vi "Exit Initialize (User).vi"(8 "error in":errorcluster, 11 "Node in":refnum<class "BLS Cycler Template.lvclass">) -> (0 "error out":errorcluster, 3 "Node out":refnum<class "BLS Cycler Template.lvclass">)   [LabVIEW 2023, in "BLS Cycler Template.lvlib" / "BLS Cycler Template.lvclass"]
uses:
  BLS Cycler Template.lvclass
  BLS Cycler Template.lvclass/BLS Cycler Template.ctl
  bls-capabilities/src/Capabilities/High Level Capabilities/Cycler/Cycler.lvclass
  <vilib>/ADAS Replay HIL/Template Node/Plugin/Template Node/Template Node.lvclass
  C:/Program Files/National Instruments/LabVIEW 2023/vi.lib/ADAS Replay HIL/Template Node/Plugin/Template Node/Template Node.lvclass
  C:/Program Files/National Instruments/ADAS Replay HIL/EVO SDK/Linux RT/evoLabVIEWAPI/evoBlockPlugin.lvlibp/evoBlockPlugin/BlockPluginInterface.2020.1/BlockPluginInterface.2020.1.lvclass
  C:/Users/amomin/BLS/bls-cycler-plugin-template/src/Plugin/BLS Cycler Template/BLS Cycler Template.lvclass
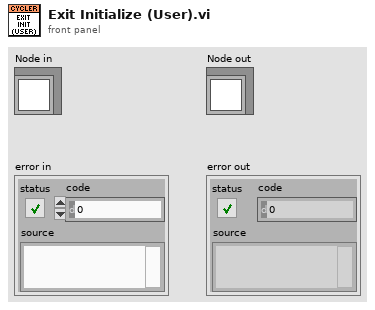
[diagram p1: front panel]
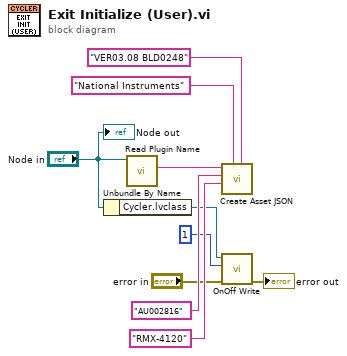
[diagram p0: block diagram]
diagram:
  n1 = Unbundle By Name("Node in") -> ("Cycler.lvclass"=w1:refnum<class "Cycler.lvclass">)
  n2 = call <vilib>:"Read Plugin Name.vi"("Template Node in"="Node in") -> ("Plugin Name"=w10:string)  [unwired: 8 in, 2 out]
  n3 = call "Create Asset JSON.vi"("firmwareVersion"="VER03.08 BLD0248", "vendorName"="National Instruments", "modelName"="RMX-4120", "serialNumber"="AU002816", "pluginName"=w10) -> ()  [unwired: 5 in, 2 out]
  n4 = call "OnOff Write.vi"("error in"="error in", "OnOff STS"=1, "Cycler in"=w1) -> ("error out"=→"error out":errorcluster)  [unwired: 7 in, 1 out]
  "Node out" <- "Node in"
